vi "Test Method Template 1.vi"(11 "Test Case In":refnum<class "My Test.lvclass">) -> (0 "error out":errorcluster, 3 "Test Case Out":refnum<class "My Test.lvclass">)   [LabVIEW 2020, in "My Test.lvclass"]
uses:
  My Test.lvclass
  C:/Program Files/National Instruments/LabVIEW 2026/vi.lib/Astemes/LUnit/Test Case.lvclass
  <vilib>/Astemes/LUnit/Test Case.lvclass/Test Case.ctl
  My Test.lvclass/My Test.ctl
  4993e8ee-a06a-463a-9684-69129f64d5ce.vi
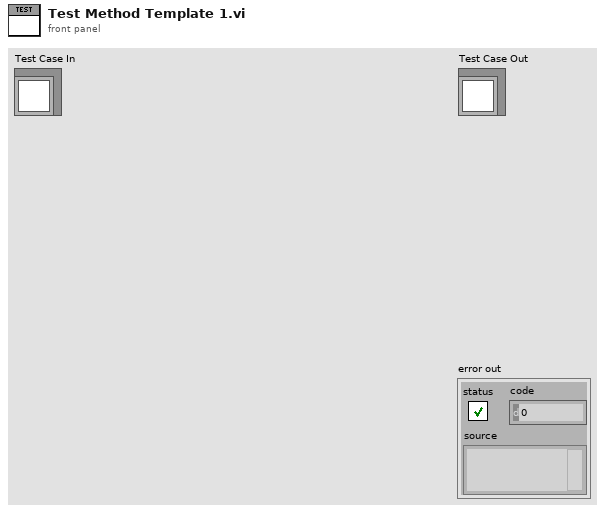
[diagram p1: front panel]
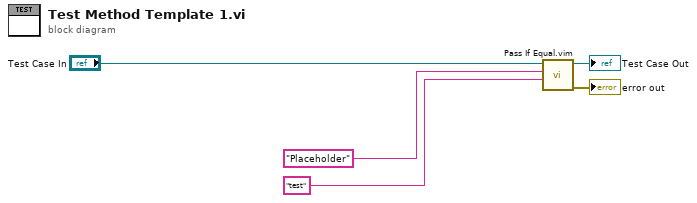
[diagram p0: block diagram]
diagram:
  n1 = call "Pass If Equal.vim"("Actual"="test", "Expected"="Placeholder", "LUnit Test Case In"="Test Case In") -> ("error out"=→"error out":errorcluster, "LUnit Test Case Out"=→"Test Case Out":refnum<class "My Test.lvclass">)  [unwired: 7 in]
